vi "Initialize Tag.vi"(4 "Log":bool, 6 "Units":string, 7 "Keyword":string, 8 "error in (no error)":errorcluster, 9 "Data Type":string(combo), 10 "Tag Name":string, 11 "Logger in.lvclass":refnum<class "Logger.lvclass">) -> (0 "error out":errorcluster, 3 "Logger out.lvclass":refnum<class "Logger.lvclass">)   [LabVIEW 2019, in "Logger.lvclass"]
uses:
  Logger.lvclass
  Logger.lvclass/Logger.ctl
  <vilib>/Skyline/Tag/Wrapper/Wrapper_class/NI Skyline Tag.lvclass
  <vilib>/Skyline/Tag/Shared/typedefs/TagProperty.ctl
  <vilib>/Skyline/Configuration/Configuration HTTP_class/NI Skyline Configuration HTTP.lvclass
  <vilib>/Skyline/Tag/Shared/typedefs/DataType.ctl
  <vilib>/Skyline/Tag/Wrapper/Wrapper HTTP_class/Open Tag HTTP.vi
  <vilib>/Skyline/Tag/Shared/NI Skyline Tag.lvlib
  <vilib>/Skyline/Tag/Wrapper/Wrapper HTTP_class/NI Skyline Tag HTTP.lvclass
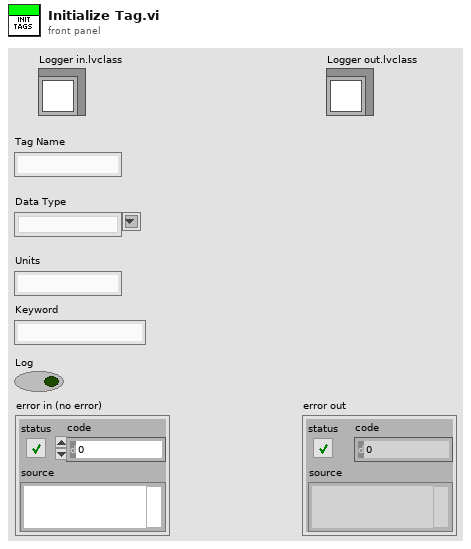
[diagram p1: front panel]
types:
  T1 = cluster{"Tag Units":string, "Tag Path":string, "Waveform":waveform(dbl), "Log":bool, "Tag Reference":refnum<class "NI Skyline Tag.lvclass">}
  T2 = typedef "NI Skyline Tag.lvlib/DataType.ctl" = enum32{"Double", "I32", "String", "Boolean", "U64", "Timestamp"}
  T3 = typedef "NI Skyline Tag.lvlib/TagProperty.ctl" = cluster{"key":string, "value":string}
  T4 = cluster{"Tag Units":string, "Tag Path":string, "Waveform":waveform(dbl), "Log":bool, "Tag Reference":refnum<class "NI Skyline Tag.lvclass">}[]
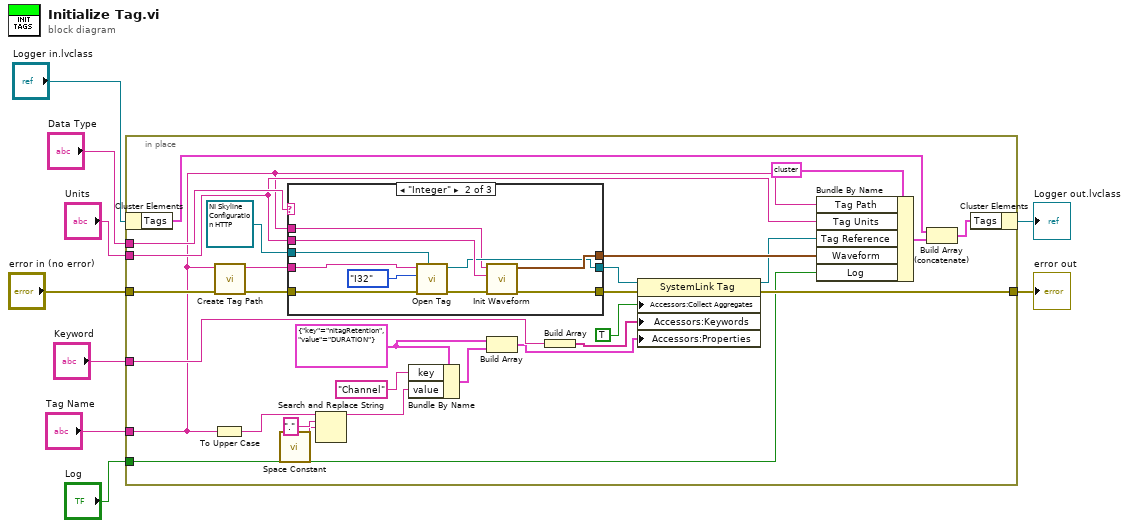
[diagram p0: block diagram]
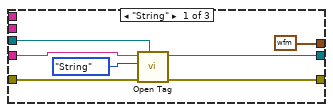
[diagram p2: hidden frame]
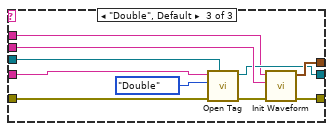
[diagram p3: hidden frame]
diagram:
  n1 = in-place {
    in-place-border: [w27] -> w9
    in-place-border: "Tag Name" -> [w11]
    in-place-border: "Data Type" -> [w37]
    in-place-border: "Units" -> [w36]
    in-place-border: "error in (no error)" -> [w22]
    in-place-border: "Keyword" -> [w24]
    in-place-border: "Log" -> [w20]
    w18 = T3 {"key"="nitagRetention", "value"="DURATION"} ("Property")
    n2 = in-place-cluster #1("Logger in.lvclass") -> ("Tags"=w33:T4)
    n3 = To Upper Case(1:w11) -> (0:w15:string)
    n4 = call "Create Tag Path.vi"("error in (no error)"=w22, "tag name"=w11) -> ("error out"=w21:errorcluster, "path"=w34:string)  [unwired: 8 in]
    n5 = call <vilib>:"Space Constant.vi"() -> ("String"=w13:string)
    n6 = case shown="\"Integer\"" w37 {
      tunnel: [w41 w54 w64] -> w28
      tunnel: [w42 w48 w58] -> w26
      tunnel: w36 -> [_ w52 w62]
      tunnel: [waveform(dbl) {"t0"=timestamp(0 s since 1904-01-01), "dt"=1.0, "Y"=[]} ("waveform") w53 w63] -> w35
      tunnel: w34 -> [w40 w50 w59]
      tunnel: w21 -> [w43 w51 w61]
      tunnel: w11 -> [_ w46 w56]
      tunnel: refnum<class "NI Skyline Configuration HTTP.lvclass"> refnum ("configuration") -> [w38 w45 w55]
      frame "String" {
        n7 = call-poly <vilib>:"Open Tag.vi"("configuration"=w38, "error in (no error)"=w43, "Data Type"=DataType."String", "path"=w40) -> ("error out"=w41:errorcluster, "tag"=w42:refnum<class "NI Skyline Tag.lvclass">)  [unwired: 6 in]
      }
      frame "Integer" {
        n8 = call-poly <vilib>:"Open Tag.vi"("configuration"=w45, "error in (no error)"=w51, "Data Type"=DataType."I32" ("data type"), "path"=w50) -> ("error out"=w49:errorcluster, "tag"=w48:refnum<class "NI Skyline Tag.lvclass">)  [unwired: 6 in]
        n9 = call "Init Waveform.vi"("error in (no error)"=w49, "Units"=w52, "Tag Name"=w46) -> ("error out"=w54:errorcluster, "waveform"=w53:waveform(dbl))  [unwired: 7 in]
      }
      frame "Double", Default {
        n10 = call-poly <vilib>:"Open Tag.vi"("configuration"=w55, "error in (no error)"=w61, "Data Type"=DataType."Double", "path"=w59) -> ("error out"=w57:errorcluster, "tag"=w58:refnum<class "NI Skyline Tag.lvclass">)  [unwired: 6 in]
        n11 = call "Init Waveform.vi"("error in (no error)"=w57, "Units"=w62, "Tag Name"=w56) -> ("error out"=w64:errorcluster, "waveform"=w63:waveform(dbl))  [unwired: 7 in]
      }
    }
    n12 = Search and Replace String(input string=w15, search string=".", replace string=w13) -> (result string=w12:string)  [unwired: 5 in, 3 out]
    n13 = Bundle By Name(cluster=w18, "key"="Channel", "value"=w12) -> (w17:T3)
    n14 = Build Array(w18, w17) -> (w19:T3[])
    n15 = Build Array(w24) -> (w23:string[])
    n16 = property class="SystemLink Tag"(reference=w26, error in=w28, "Accessors:Collect Aggregates"=TRUE ("Collect Aggregates"), "Accessors:Keywords"=w23, "Accessors:Properties"=w19) -> (reference out=w25:refnum<class "NI Skyline Tag.lvclass">, error out=w27:errorcluster)
    n17 = Bundle By Name(cluster=T1 {"Tag Units"="", "Tag Path"="", "Waveform"={"t0"=timestamp(0 s since 1904-01-01), "dt"=1.0, "Y"=[]}, "Log"=FALSE, "Tag Reference"=refnum} ("Tag"), "Tag Path"=w11, "Tag Units"=w36, "Tag Reference"=w25, "Waveform"=w35, "Log"=w20) -> (w31:T1)
    n18 = Build Array (concatenate)(w33, w31) -> (w32:T4)
    n19 = in-place-cluster #1("Tags"=w32) -> (→"Logger out.lvclass":refnum<class "Logger.lvclass">)
  }
  "error out" <- w9
